vi "Calc Dev (Netway).vi"(0 "Verify Table IN":string[][](array[string]), 1 "Units":T2, 2 "Channel to Cal":T1=enum."AIO5", 5 "Dev Table 1 Ref":refnum<vi>) -> (14 "Verify Table OUT":string[][](array[string]))   [LabVIEW 2013]
uses:
  Type Defs/Units Type Def (Netway).ctl
  Type Defs/Channel Type Def (Netway).ctl
  <vilib>/Utility/miscctls.llb/LVRowAndColumnTypeDef.ctl
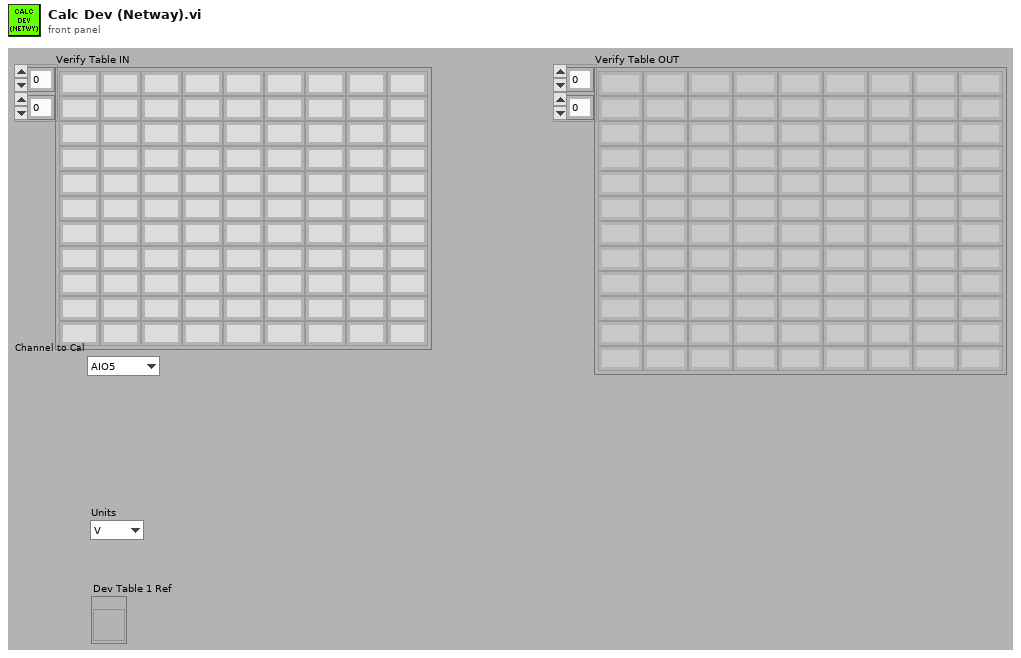
[diagram p1: front panel]
types:
  T1 = typedef "Channel Type Def (Netway).ctl" = enum16{"IO1", "IO2", "IO3", "IO4", "IO5", "IO6", "IO7", "IO8", "IO9", "IO10", "IO11", "IO12", "AIO1", "AIO2", "AIO3", "AIO4", "AIO5", "AIO6", "AIO7", "AIO8"}
  T2 = typedef "Units Type Def (Netway).ctl" = enum16{"V", "%", "Hz"}
  T3 = typedef "LVRowAndColumnTypeDef.ctl" = cluster{"Row":i32, "Column":i32}
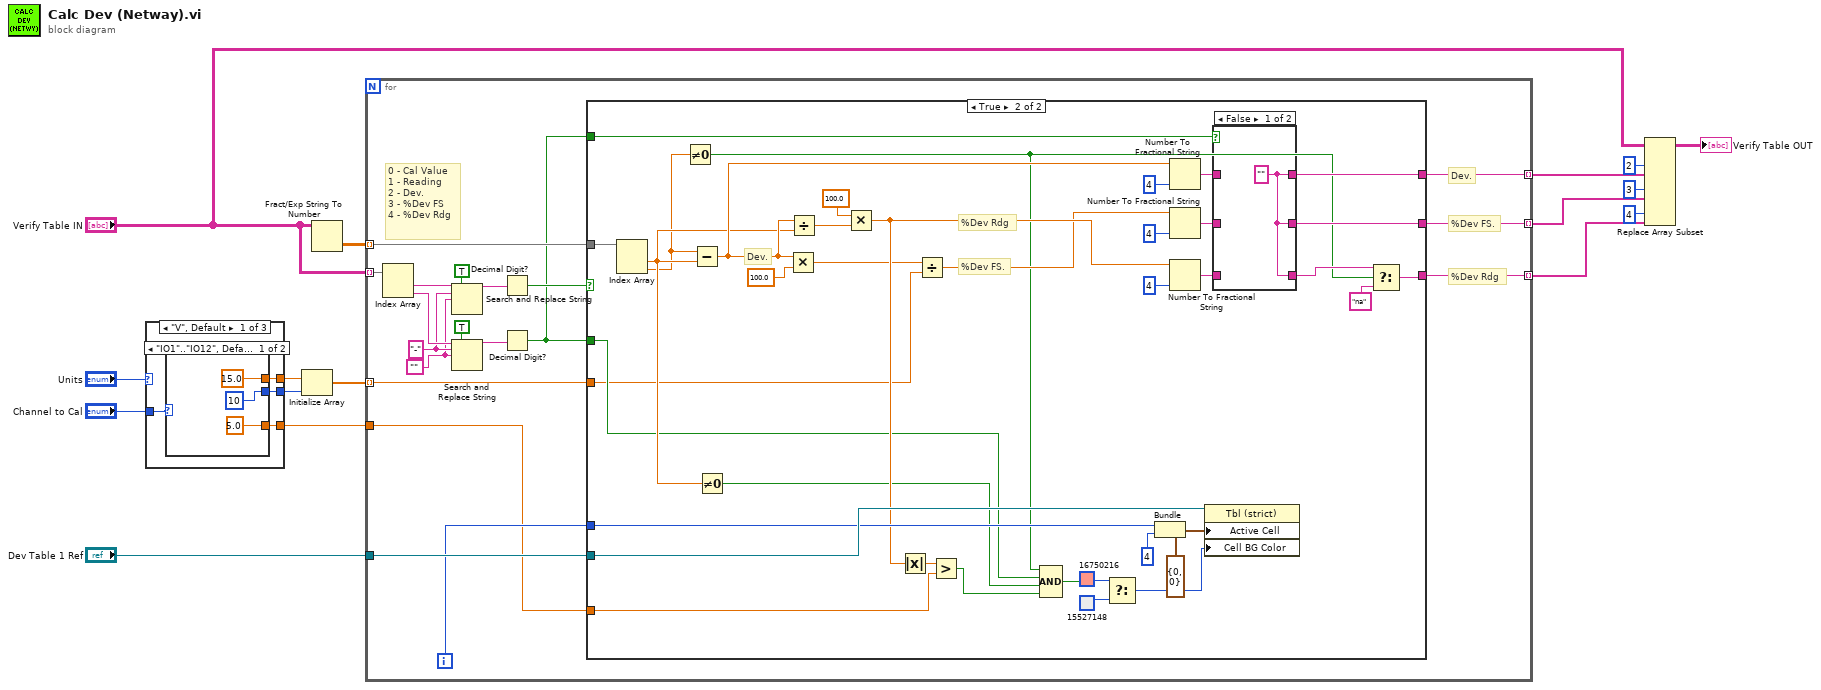
[diagram p0: block diagram]
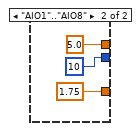
[diagram p2: hidden frame]
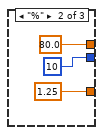
[diagram p3: hidden frame]
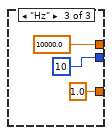
[diagram p4: hidden frame]
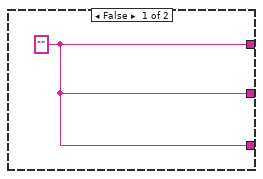
[diagram p5: hidden frame]
diagram:
  n1 = case shown="\"V\", Default" "Units" {
    tunnel: [w20 80.0 10000.0] -> w14
    tunnel: [w19 10 ("dimension size") 10 ("dimension size")] -> w13
    tunnel: [w18 1.25 ("y") 1.0 ("y")] -> w2
    tunnel: "Channel to Cal" -> [w17 _ _]
    frame "V", Default {
      n2 = case shown="\"IO1\"..\"IO12\", Default" w17 {
        tunnel: [15.0 5.0] -> w20
        tunnel: [10 ("dimension size") 10 ("dimension size")] -> w19
        tunnel: [5.0 ("y") 1.75 ("y")] -> w18
        frame "IO1".."IO12", Default {
        }
        frame "AIO1".."AIO8" {
        }
      }
    }
    frame "%" {
    }
    frame "Hz" {
    }
  }
  n3 = Initialize Array(w14, w13) -> (w10:dbl[])
  n4 = Fract/Exp String To Number(string="Verify Table IN") -> (number=w16:dbl[][])  [unwired: 3 in, 1 out]
  n5 = for {
    tunnel: w16 -> [w50] mode=indexing
    tunnel: "Verify Table IN" -> [w51] mode=indexing
    tunnel: "Dev Table 1 Ref" -> [w49]
    tunnel: w10 -> [w45] mode=indexing
    tunnel: [w44] -> w7 mode=indexing
    tunnel: [w43] -> w6 mode=indexing
    tunnel: [w42] -> w5 mode=indexing
    tunnel: w2 -> [w33]
    i -> [w48]
    w34 = ""
    w35 = "-" ("search string")
    # "%Dev Rdg"
    # "%Dev FS."
    # "Dev."
    # "0 - Cal Value\n1 - Reading\n2 - Dev.\n3 - %Dev FS\n4 - %Dev Rdg"
    n6 = Index Array(array=w51) -> (element #1=w37:string, element #2=w41:string)  [unwired: 2 in]
    n7 = Search and Replace String(replace all?=TRUE ("replace all? (F)"), input string=w37, search string=w35, replace string=w34) -> (result string=w36:string)  [unwired: 4 in, 3 out]
    n8 = Search and Replace String(replace all?=TRUE ("replace all? (F)"), input string=w41, search string=w35, replace string=w34) -> (result string=w40:string)  [unwired: 4 in, 3 out]
    n9 = Decimal Digit?(1:w36) -> (0:w47:bool)
    n10 = Decimal Digit?(1:w40) -> (0:w46:bool)
    n11 = case shown="True" w47 {
      tunnel: w50 -> [_ w90]
      tunnel: [w52 w65] -> w44
      tunnel: [w52 w64] -> w43
      tunnel: [w52 w55] -> w42
      tunnel: w49 -> [_ w81]
      tunnel: w48 -> [_ w80]
      tunnel: w46 -> [_ w63]
      tunnel: w46 -> [_ w62]
      tunnel: w45 -> [_ w59]
      tunnel: w33 -> [_ w53]
      frame False {
        w52 = ""
      }
      frame True {
        # "%Dev Rdg"
        # "%Dev FS."
        # "Dev."
        n12 = Index Array(array=w90) -> (element #1=w70:dbl, element #2=w58:dbl)  [unwired: 2 in]
        n13 = Not Equal To 0?(x=w58) -> (x != 0?=w54:bool)
        n14 = Subtract(x=w58, y=w70) -> (x-y=w85:dbl)
        n15 = Not Equal To 0?(x=w70) -> (x != 0?=w69:bool)
        n16 = Multiply(x=w85, y=100.0) -> (x*y=w60:dbl)
        n17 = Divide(x=w85, y=w70) -> (x/y=w84:dbl)
        n18 = Multiply(x=100.0 ("y"), y=w84) -> (x*y=w73:dbl)
        n19 = Absolute Value(x=w73) -> (abs(x)=w82:dbl)
        n20 = Divide(x=w60, y=w59) -> (x/y=w61:dbl)
        n21 = Greater?(x=w82, y=w53) -> (0:w72:bool)
        n22 = Compound Arithmetic op=AND(w54, w62, w69, w72) -> (w71:bool)
        n23 = Select(t=u32 16750216, s=w71, f=u32 15527148) -> (s? t:f=w74:u32)
        n24 = Bundle(cluster=T3 {"Row"=0, "Column"=0} ("Active Cell:Active Cell"), "Row"=w80, "Column"=4) -> (w78:T3)
        n25 = Number To Fractional String(number=w85, precision (6)=i16 4) -> (F-format string=w68:string)  [unwired: 2 in]
        n26 = Number To Fractional String(number=w61, precision (6)=i16 4) -> (F-format string=w67:string)  [unwired: 2 in]
        n27 = Number To Fractional String(number=w73, precision (6)=i16 4) -> (F-format string=w66:string)  [unwired: 2 in]
        n28 = property on="Property Node" class="Tbl (strict)"(reference=w81, "Active Cell"=w78, "Cell BG Color"=w74) -> ()  [unwired: 1 in, 2 out]
        n29 = case shown="False" w63 {
          tunnel: [w91 w94] -> w65
          tunnel: w68 -> [_ w94]
          tunnel: w67 -> [_ w93]
          tunnel: [w91 w93] -> w64
          tunnel: w66 -> [_ w92]
          tunnel: [w91 w92] -> w56
          frame False {
            w91 = ""
          }
          frame True {
          }
        }
        n30 = Select(t=w56, s=w54, f="na") -> (s? t:f=w55:string)
      }
    }
  }
  n31 = Replace Array Subset(array="Verify Table IN", new element #1=w7, index (col) #1=2 ("disabled index (col)"), new element #2=w6, index (col) #2=3 ("disabled index (col)"), new element #3=w5, index (col) #3=4 ("disabled index (col)")) -> (→"Verify Table OUT":string[][])  [unwired: 3 in]
